vi "R5Master.vi"(6 "LabVIEW Web Service":refnum<class "Web Service.lvclass">=refnum) -> ()   [LabVIEW 2016]
uses:
  <vilib>/wsapi/Web Service.lvclass
  <vilib>/Platform/TimedLoop/XDataNode/XDataNode.xnode
  <vilib>/Platform/TimedLoop/XDataNode/nitl_modes.ctl
  <vilib>/Platform/TimedLoop/XDataNode/XDNodeRunTimeDep.lvlib
  <vilib>/Platform/TimedLoop/XDataNode/wakeup.ctl
  <vilib>/Platform/TimedLoop/XDataNode/timing_clust.ctl
  <vilib>/Platform/TimedLoop/XDataNode/loadnilvce.vi
  R5Controls/R5SBR_SetParams.ctl
  Controls/pH_SetParams Standard.ctl
panel:
  out "Probes":cluster{"Value":dbl, "Value":dbl}(graph)
  in  "R5SBRSetParams":T1
  in  "R5SBRManual":cluster{"Media Pump":bool, "Effluent Pump":bool}
  out "error out":errorcluster
  out "error out (DATA COLLECT)":errorcluster
  out "error out (SBR)":errorcluster
  in  "R5 SBR_Switch":bool
  in  "R5DOSetParams":T2={"Set Point, mg/L"=0.0, "Tolerance, mg/L"=0.05, "N2 Valve Gain"=5000.0, "Air Valve Gain"=1000.0}
  in  "R5DOManual":cluster{"Air MFC":dbl, "N2 MFC":dbl} {"Air MFC" scale=0.0..500.0; "N2 MFC" scale=0.0..500.0}
  in  "R5 DO_Switch":bool=TRUE
  out "R5DO":cluster{"Signal":dbl, "Value":dbl}={"Signal"=0.012310571769960223, "Value"=5.584491888741017}
  in  "R5 pH_Switch":bool=TRUE
  in  "R5 pH_SetParams":T3={"Set Point"=7.0, "Tolerance"=0.1, "Pump Time On, secs"=6.0}
  in  "R5pH_Manual":cluster{"Acid Pump":bool, "Base Pump":bool}
  out "pH":cluster{"Signal":dbl, "Value":dbl}={"Signal"=0.0127343038254794, "Value"=7.4567616069444576}
  out "Timestamp":string="09/22/2017 10:45:23.660"
  out "Status":string="Off"
  out "Cycle Time Elapsed":dbl
  out "Phase Time Elapsed":dbl
  # "Use the web service input terminal to call the VIs on the Service subpalette of the Web Services palette. Do not remove it from the connector pane unless you don't need access to the palette."
  # "Any additional terminals added to the connector pane of a startup VI will be ignored."
  # "DO Control"
  # "SBR Control"
  # "pH Control"
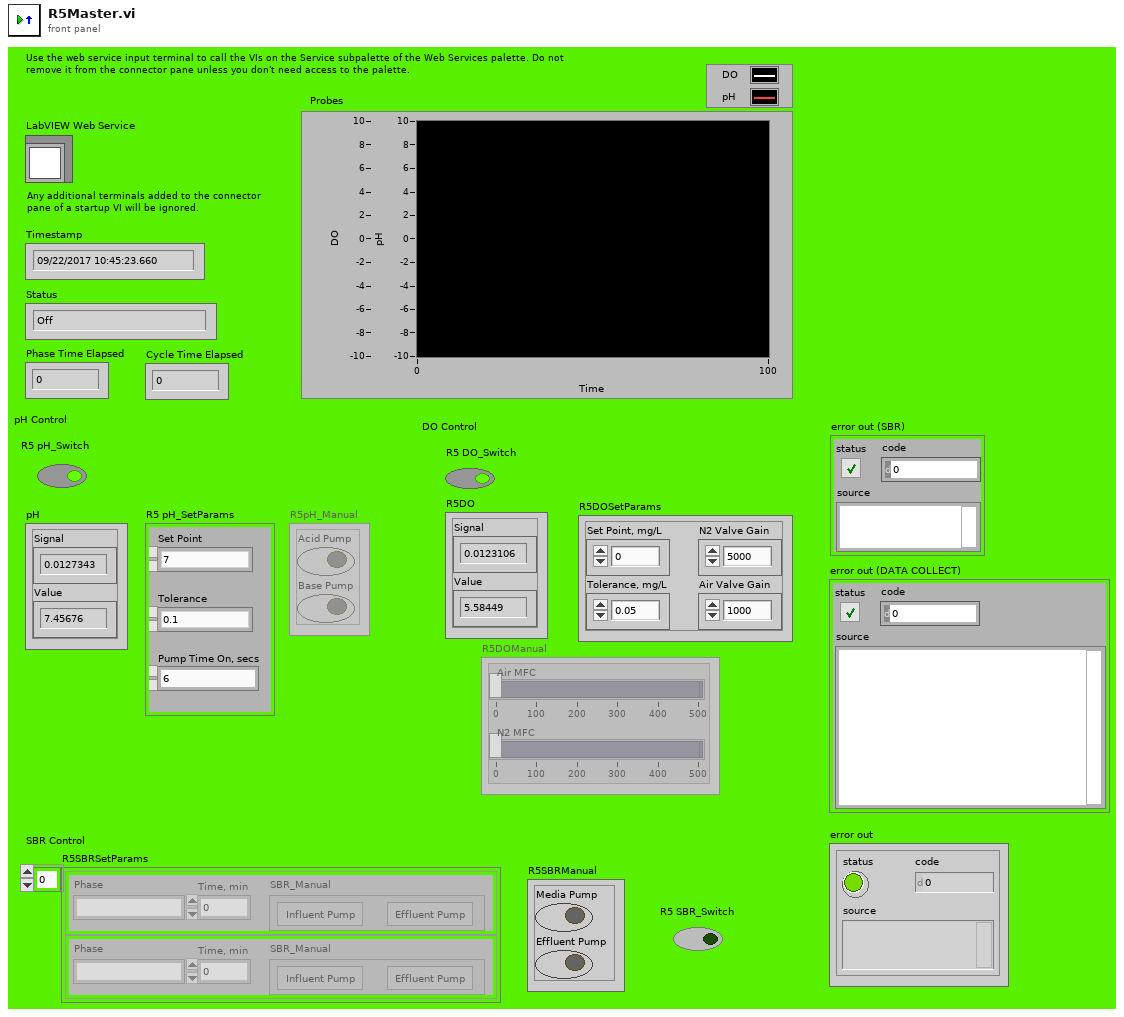
[diagram p1: front panel]
types:
  T1 = typedef "R5SBR_SetParams.ctl" = cluster{"Phase":string, "Time, min":dbl, "SBR_Manual":cluster{"Influent Pump":bool, "Effluent Pump":bool}}[]
  T2 = cluster{"Set Point, mg/L":dbl, "Tolerance, mg/L":dbl, "N2 Valve Gain":dbl, "Air Valve Gain":dbl}
  T3 = typedef "pH_SetParams Standard.ctl" = cluster{"Set Point":dbl, "Tolerance":dbl, "Pump Time On, secs":dbl}
  T4 = typedef "XDNodeRunTimeDep.lvlib/timing_clust.ctl" = cluster{"Expected End [f-1]":u64, "Actual End [f-1]":u64, "Finished Late? [f-1]":bool, "Expected End [i-1]":u64, "Actual End [i-1]":u64, "Finished Late? [i-1]":bool, "Expected Start [i]":u64, "Actual Start [i]":u64, "Expected Start [f]":u64, "Actual Start [f]":u64, "Source Name":string, "Structure Name":string, "Period":i64, "Deadline":i64, "Offset":i64, "Start":i64, "Priority":i32, "Timeout":i32, "Mode":T5, "Wakeup Reason":T6, "Error":errorcluster, "Source Type":string, "Secondary Source Type":string, "Global End Time":u64, "Global Start Time":u64, "Frame Duration":u64, "Iteration Duration":u64, "Assigned CPU":i32, "I/O Scan Engine Mode":u32}
  T5 = typedef "XDNodeRunTimeDep.lvlib/nitl_modes.ctl" = enum32{"No Change", "Process missed periods, maintain original phase", "Discard missed periods, maintain original phase", "Process missed periods, ignore original phase", "Discard missed periods, ignore original phase"}
  T6 = typedef "XDNodeRunTimeDep.lvlib/wakeup.ctl" = enum32{"Normal", "Aborted", "Asynchronous wakeup", "Timing source error", "Timed loop error", "Timeout"}
  T7 = enum8{"Enabled", "Disabled", "Disabled and Grayed Out"}
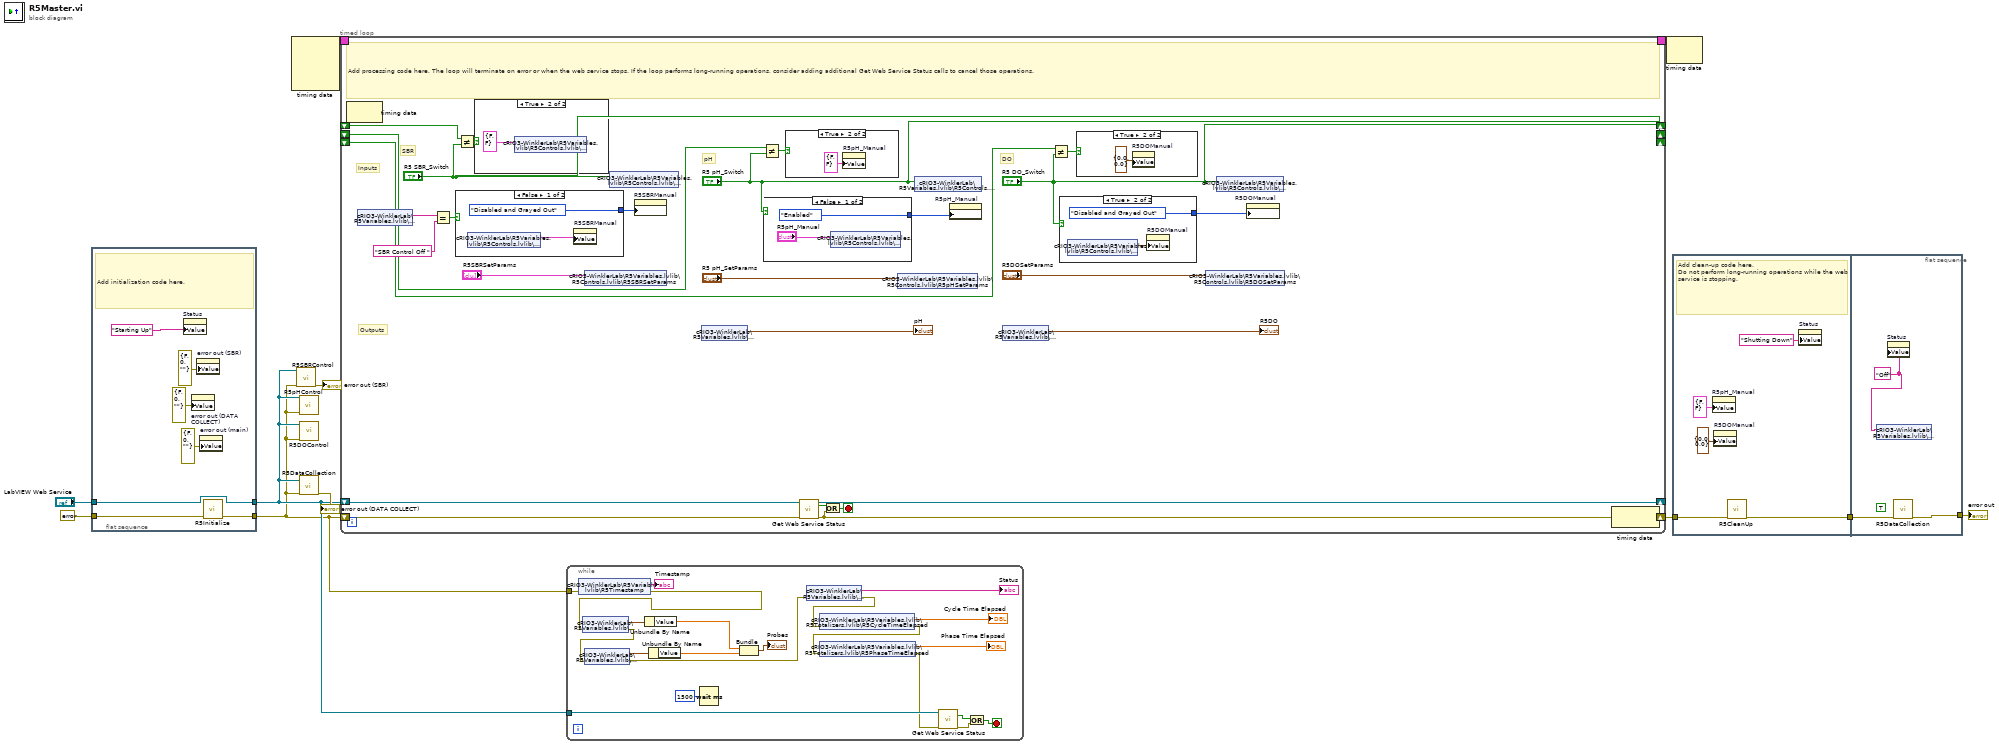
[diagram p0: block diagram]
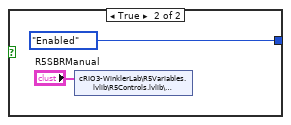
[diagram p5: hidden frame]
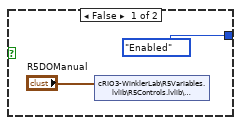
[diagram p6: hidden frame]
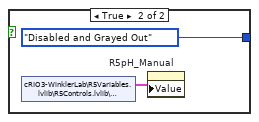
[diagram p7: hidden frame]
diagram:
  n1 = flat-sequence {
    tunnel: "LabVIEW Web Service" -> [w18]
    tunnel: errorcluster {"status"=FALSE, "code"=0, "source"=""} ("error constant") -> [w12]
    tunnel: [w13] -> w1
    tunnel: [w18] -> w2
    frame #0 {
      # "Add initialization code here."
      n2 = property on="Status" class="Str"("Value"="Starting Up" ("Status")) -> ()  [unwired: 2 in, 2 out]
      n3 = property on="error out (DATA COLLECT)" class="Clust (strict)"("Value"=errorcluster {"status"=FALSE, "code"=0, "source"=""} ("error out (DATA COLLECT)")) -> ()  [unwired: 2 in, 2 out]
      n4 = property on="error out (SBR)" class="Clust (strict)"("Value"=errorcluster {"status"=FALSE, "code"=0, "source"=""} ("error out (SBR)")) -> ()  [unwired: 2 in, 2 out]
      n5 = property on="error out (main)" class="Clust (strict)"("Value"=errorcluster {"status"=FALSE, "code"=0, "source"=""} ("error out")) -> ()  [unwired: 2 in, 2 out]
      n6 = call "R5Initialize.vi"("error in (no error)"=w12) -> ("error out"=w13:errorcluster)  [unwired: 10 in]
    }
  }
  n7 = node-c288() -> (w8:T4)  [unwired: 4 in]
  n8 = call "R5SBRControl.vi"("error constant"=w1, "LabVIEW Web Service"=w2) -> ("error out"=→"error out (SBR)":errorcluster)  [unwired: 9 in]
  n9 = call "R5pHControl.vi"("error constant"=w1, "LabVIEW Web Service"=w2) -> ()  [unwired: 10 in]
  n10 = call "R5DataCollection.vi"("error constant"=w1, "LabVIEW Web Service"=w2) -> ("error out"=→"error out (DATA COLLECT)":errorcluster)  [unwired: 9 in]
  n11 = call "R5DOControl.vi"("error constant"=w1, "LabVIEW Web Service"=w2) -> ()  [unwired: 10 in]
  n12 = timed-loop {
    shift-right: [w42] -> w9
    shift-left: w1 -> [w41]
    shift-right: [w39] -> _
    shift-left: w2 -> [w39]
    timing: w8 -> [_]
    timing-out: [_] -> w7
    shift-right: ["R5 SBR_Switch"] -> _
    shift-left: _ -> [w29]
    shift-right: ["R5 pH_Switch"] -> _
    shift-left: _ -> [w35]
    shift-right: ["R5 DO_Switch"] -> _
    shift-left: _ -> [w33]
    stop <- w40 stop-if-true
    # "DO"
    # "pH"
    # "Outputs"
    # "Inputs"
    # "SBR"
    # "Add processing code here. The loop will terminate on error or when the web service stops. If the loop performs long-running operations, consider adding additional Get Web Service Status calls to cancel those operations."
    n13 = node-c288() -> ()  [unwired: 1 in, 1 out]
    n14 = shared-variable "cRIO3-WinklerLab\\R5Variables.lvlib\\R5Status"() -> (w28:string)  [unwired: 1 in, 1 out]
    n15 = Equal?(x=w28, y="SBR Control Off " ("string")) -> (x = y?=w30:bool)
    n16 = case shown="False" w30 {
      tunnel: [T7."Disabled and Grayed Out" ("Disabled") T7."Enabled" ("Disabled")] -> w19
      frame False {
        n17 = shared-variable "cRIO3-WinklerLab\\R5Variables.lvlib\\R5Controls.lvlib\\R5SBRManual"() -> (w47:cluster{"Media Pump":bool, "Effluent Pump":bool})  [unwired: 1 in, 1 out]
        n18 = property on="R5SBRManual" class="Clust (strict)"("Value"=w47) -> ()  [unwired: 2 in, 2 out]
      }
      frame True {
        n19 = shared-variable "cRIO3-WinklerLab\\R5Variables.lvlib\\R5Controls.lvlib\\R5SBRManual"("R5SBRManual") -> ()  [unwired: 1 in, 1 out]
      }
    }
    n20 = Not Equal?(x=w29, y="R5 SBR_Switch") -> (x != y?=w36:bool)
    n21 = case shown="True" w36 {
      frame False {
      }
      frame True {
        n22 = shared-variable "cRIO3-WinklerLab\\R5Variables.lvlib\\R5Controls.lvlib\\R5SBRManual"(cluster{"Media Pump":bool, "Effluent Pump":bool} {"Media Pump"=FALSE, "Effluent Pump"=FALSE} ("R5SBRManual")) -> ()  [unwired: 1 in, 1 out]
      }
    }
    n23 = shared-variable "cRIO3-WinklerLab\\R5Variables.lvlib\\R5Controls.lvlib\\R5SBRSetParams"("R5SBRSetParams") -> ()  [unwired: 1 in, 1 out]
    n24 = shared-variable "cRIO3-WinklerLab\\R5Variables.lvlib\\R5Controls.lvlib\\R5SBRSwitch"("R5 SBR_Switch") -> ()  [unwired: 1 in, 1 out]
    n25 = property on="R5SBRManual" class="Clust (strict)"("DisabledEnum"=w19) -> ()  [unwired: 2 in, 2 out]
    n26 = shared-variable "cRIO3-WinklerLab\\R5Variables.lvlib\\R5Signals.lvlib\\R5pH"() -> (→"pH":cluster{"Signal":dbl, "Value":dbl})  [unwired: 1 in, 1 out]
    n27 = Not Equal?(x=w35, y="R5 pH_Switch") -> (x != y?=w34:bool)
    n28 = case shown="False" "R5 pH_Switch" {
      tunnel: [T7."Enabled" ("Disabled") T7."Disabled and Grayed Out" ("Disabled")] -> w38
      frame False {
        n29 = shared-variable "cRIO3-WinklerLab\\R5Variables.lvlib\\R5Controls.lvlib\\R5pHManual"("R5pH_Manual") -> ()  [unwired: 1 in, 1 out]
      }
      frame True {
        n30 = shared-variable "cRIO3-WinklerLab\\R5Variables.lvlib\\R5Controls.lvlib\\R5pHManual"() -> (w57:cluster{"Acid Pump":bool, "Base Pump":bool})  [unwired: 1 in, 1 out]
        n31 = property on="R5pH_Manual" class="Clust (strict)"("Value"=w57) -> ()  [unwired: 2 in, 2 out]
      }
    }
    n32 = case shown="True" w34 {
      frame False {
      }
      frame True {
        n33 = property on="R5pH_Manual" class="Clust (strict)"("Value"=cluster{"Acid Pump":bool, "Base Pump":bool} {"Acid Pump"=FALSE, "Base Pump"=FALSE} ("R1pH_Manual")) -> ()  [unwired: 2 in, 2 out]
      }
    }
    n34 = call <vilib>:"Get Web Service Status.vi"("LabVIEW Web Service"=w39, "error in (no error)"=w41) -> ("service stopping?"=w43:bool, "error out"=w42:errorcluster)  [unwired: 11 in, 1 out]
    n35 = Or(x=w43, y=w42) -> (x .or. y?=w40:bool)
    n36 = shared-variable "cRIO3-WinklerLab\\R5Variables.lvlib\\R5Controls.lvlib\\R5pHSetParams"("R5 pH_SetParams") -> ()  [unwired: 1 in, 1 out]
    n37 = shared-variable "cRIO3-WinklerLab\\R5Variables.lvlib\\R5Controls.lvlib\\R5pHSwitch"("R5 pH_Switch") -> ()  [unwired: 1 in, 1 out]
    n38 = property on="R5pH_Manual" class="Clust (strict)"("DisabledEnum"=w38) -> ()  [unwired: 2 in, 2 out]
    n39 = shared-variable "cRIO3-WinklerLab\\R5Variables.lvlib\\R5Signals.lvlib\\R5DO"() -> (→"R5DO":cluster{"Signal":dbl, "Value":dbl})  [unwired: 1 in, 1 out]
    n40 = Not Equal?(x=w33, y="R5 DO_Switch") -> (x != y?=w32:bool)
    n41 = case shown="True" "R5 DO_Switch" {
      tunnel: [T7."Enabled" ("Disabled") T7."Disabled and Grayed Out" ("Disabled")] -> w37
      frame False {
        n42 = shared-variable "cRIO3-WinklerLab\\R5Variables.lvlib\\R5Controls.lvlib\\R5DOManual"("R5DOManual") -> ()  [unwired: 1 in, 1 out]
      }
      frame True {
        n43 = shared-variable "cRIO3-WinklerLab\\R5Variables.lvlib\\R5Controls.lvlib\\R5DOManual"() -> (w53:cluster{"Air MFC":dbl, "N2 MFC":dbl})  [unwired: 1 in, 1 out]
        n44 = property on="R5DOManual" class="Clust (strict)"("Value"=w53) -> ()  [unwired: 2 in, 2 out]
      }
    }
    n45 = case shown="True" w32 {
      frame False {
      }
      frame True {
        n46 = property on="R5DOManual" class="Clust (strict)"("Value"=cluster{"Air MFC":dbl, "N2 MFC":dbl} {"Air MFC"=0.0, "N2 MFC"=0.0} ("R1DOManual")) -> ()  [unwired: 2 in, 2 out]
      }
    }
    n47 = shared-variable "cRIO3-WinklerLab\\R5Variables.lvlib\\R5Controls.lvlib\\R5DOSetParams"("R5DOSetParams") -> ()  [unwired: 1 in, 1 out]
    n48 = shared-variable "cRIO3-WinklerLab\\R5Variables.lvlib\\R5Controls.lvlib\\R5DOSwitch"("R5 DO_Switch") -> ()  [unwired: 1 in, 1 out]
    n49 = property on="R5DOManual" class="Clust (strict)"("DisabledEnum"=w37) -> ()  [unwired: 2 in, 2 out]
    n50 = node-c288() -> ()  [unwired: 1 in, 1 out]
  }
  n51 = while {
    tunnel: w2 -> [w80]
    tunnel: w1 -> [w74]
    stop <- w77 stop-if-true
    n52 = shared-variable "cRIO3-WinklerLab\\R5Variables.lvlib\\R5Timestamp"(error in=w74) -> (→"Timestamp":string, error out=w67:errorcluster)
    n53 = shared-variable "cRIO3-WinklerLab\\R5Variables.lvlib\\R5Signals.lvlib\\R5DO"(error in=w67) -> (w69:cluster{"Signal":dbl, "Value":dbl}, error out=w68:errorcluster)
    n54 = shared-variable "cRIO3-WinklerLab\\R5Variables.lvlib\\R5Signals.lvlib\\R5pH"(error in=w68) -> (w71:cluster{"Signal":dbl, "Value":dbl}, error out=w70:errorcluster)
    n55 = Unbundle By Name(w69) -> ("Value"=w81:dbl)
    n56 = Unbundle By Name(w71) -> ("Value"=w75:dbl)
    n57 = Wait (ms)(milliseconds to wait=u32 1500) -> ()  [unwired: 1 out]
    n58 = Bundle("Value"=w81, "Value"=w75) -> (→"Probes":cluster{"Value":dbl, "Value":dbl})  [unwired: 1 in]
    n59 = shared-variable "cRIO3-WinklerLab\\R5Variables.lvlib\\R5Status"(error in=w70) -> (→"Status":string, error out=w66:errorcluster)
    n60 = shared-variable "cRIO3-WinklerLab\\R5Variables.lvlib\\R5Totalizers.lvlib\\R5CycleTimeElapsed"(error in=w66) -> (→"Cycle Time Elapsed":dbl, error out=w62:errorcluster)
    n61 = shared-variable "cRIO3-WinklerLab\\R5Variables.lvlib\\R5Totalizers.lvlib\\R5PhaseTimeElapsed"(error in=w62) -> (→"Phase Time Elapsed":dbl, error out=w63:errorcluster)
    n62 = call <vilib>:"Get Web Service Status.vi"("LabVIEW Web Service"=w80, "error in (no error)"=w63) -> ("service stopping?"=w79:bool, "error out"=w78:errorcluster)  [unwired: 11 in, 1 out]
    n63 = Or(x=w79, y=w78) -> (x .or. y?=w77:bool)
  }
  n64 = node-c288(w7) -> ()  [unwired: 1 out]
  n65 = flat-sequence {
    tunnel: w9 -> [w82]
    tunnel: [w83] -> w6
    tunnel: w6 -> [w88]
    tunnel: [w87] -> w5
    frame #0 {
      # "Add clean-up code here.\nDo not perform long-running operations while the web service is stopping."
      n66 = property on="R5pH_Manual" class="Clust (strict)"("Value"=cluster{"Acid Pump":bool, "Base Pump":bool} {"Acid Pump"=FALSE, "Base Pump"=FALSE} ("R1pH_Manual")) -> ()  [unwired: 2 in, 2 out]
      n67 = property on="R5DOManual" class="Clust (strict)"("Value"=cluster{"Air MFC":dbl, "N2 MFC":dbl} {"Air MFC"=0.0, "N2 MFC"=0.0} ("R1DOManual")) -> ()  [unwired: 2 in, 2 out]
      n68 = call "R5CleanUp.vi"("error in (no error)"=w82) -> ("error out"=w83:errorcluster)  [unwired: 10 in]
      n69 = property on="Status" class="Str"("Value"="Shutting Down" ("Status")) -> ()  [unwired: 2 in, 2 out]
    }
    frame #1 {
      w89 = "Off" ("Status")
      (unwired) TRUE ("Write Once")
      n70 = shared-variable "cRIO3-WinklerLab\\R5Variables.lvlib\\R5Status"(w89) -> ()  [unwired: 1 in, 1 out]
      n71 = property on="Status" class="Str"("Value"=w89) -> ()  [unwired: 2 in, 2 out]
      n72 = call "R5DataCollection.vi"("error constant"=w88) -> ("error out"=w87:errorcluster)  [unwired: 10 in]
    }
  }
  "error out" <- w5
